vi "id参数转换.vi"(11 "id":u16) -> (3 "table输出":string, 5 "数组资源索引":i32)   [LabVIEW 2016, in "斯坦道总氮.lvlib"]
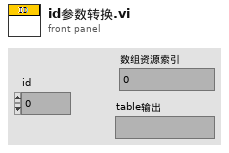
[diagram p1: front panel]
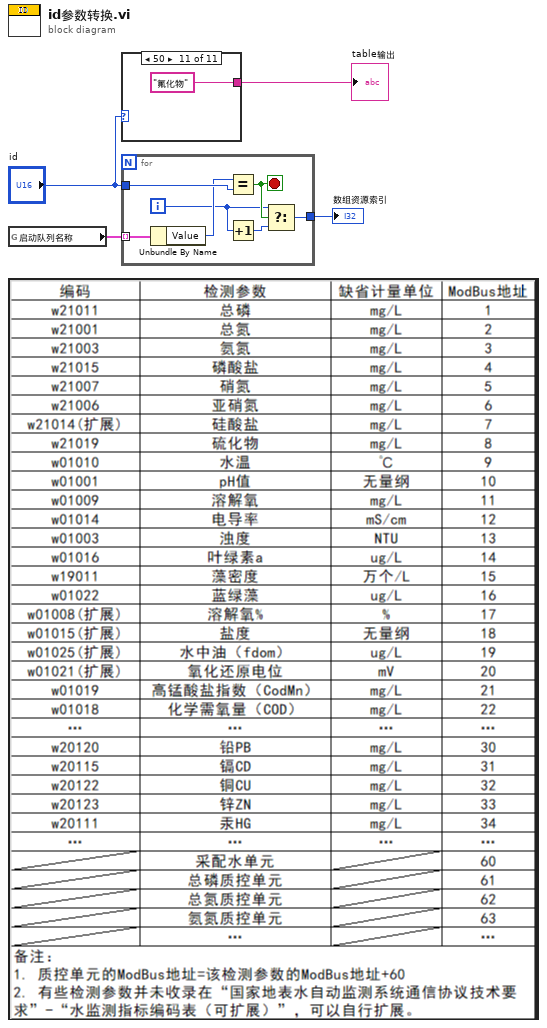
[diagram p0: block diagram]
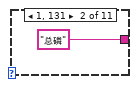
[diagram p3: hidden frame]
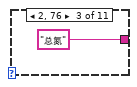
[diagram p4: hidden frame]
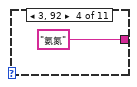
[diagram p5: hidden frame]
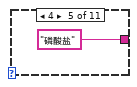
[diagram p6: hidden frame]
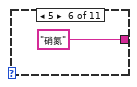
[diagram p7: hidden frame]
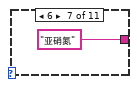
[diagram p8: hidden frame]
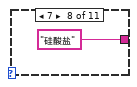
[diagram p9: hidden frame]
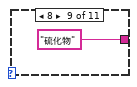
[diagram p10: hidden frame]
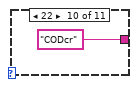
[diagram p11: hidden frame]
diagram:
  n1 = global read "model config var.vi" "启动队列名称"() -> (w3:cluster{"String":string, "Value":u16}[])
  n2 = case shown="50" "id" {
    tunnel: [_ "总磷" ("table输入") "总氮" ("table输入") "氨氮" ("table输入") "磷酸盐" ("table输入") "硝氮" ("table输入") "亚硝氮" ("table输入") "硅酸盐" ("table输入") "硫化物" ("table输入") "CODcr" ("table输入") "氟化物" ("table输入")] -> w4
    frame 0, Default {
    }
    frame 1, 131 {
    }
    frame 2, 76 {
    }
    frame 3, 92 {
    }
    frame 4 {
    }
    frame 5 {
    }
    frame 6 {
    }
    frame 7 {
    }
    frame 8 {
    }
    frame 22 {
    }
    frame 50 {
    }
  }
  "table输出" <- w4
  n3 = for {
    tunnel: w3 -> [w21] mode=indexing
    tunnel: "id" -> [w20]
    tunnel: [w15] -> w1
    i -> [w16]
    stop <- w18 stop-if-true
    n4 = Unbundle By Name(w21) -> ("Value"=w19:u16)
    n5 = Equal?(x=w19, y=w20) -> (x = y?=w18:bool)
    n6 = Increment(x=w16) -> (x+1=w17:i32)
    n7 = Select(t=w16, s=w18, f=w17) -> (s? t:f=w15:i32)
  }
  "数组资源索引" <- w1
